vi "Simulation XY update.vi"() -> ()   [LabVIEW 2013]
uses:
  subvi/simulator/Global Variables.vi
panel:
  out "Y Position":dbl
  out "X Position":dbl
  in  "stop":bool
  in  "Update Delay":u32=250
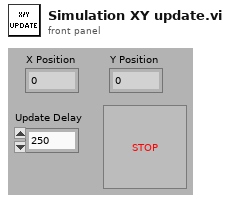
[diagram p1: front panel]
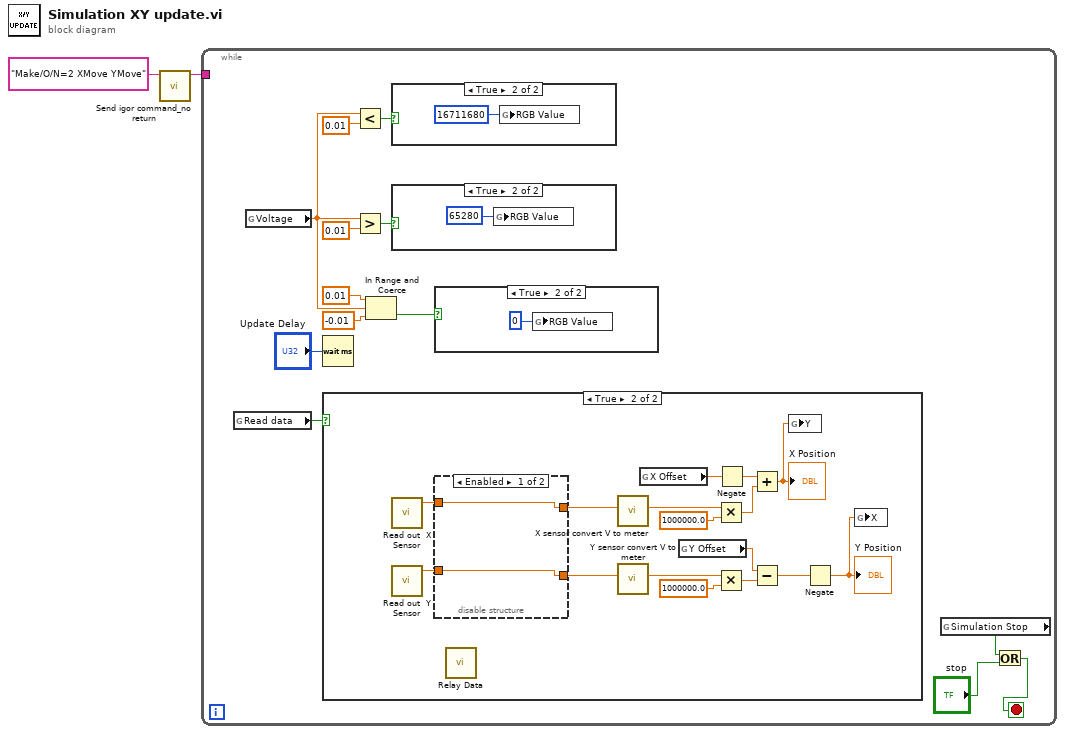
[diagram p0: block diagram]
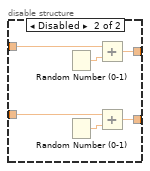
[diagram p6: hidden frame]
diagram:
  n1 = call "Send igor command_no return.vi"("Command"="Make/O/N=2 XMove YMove") -> ("History"=w1:string)  [unwired: 10 out]
  n2 = while {
    tunnel: w1 -> [_]
    stop <- w3 stop-if-true
    n3 = global read "Global Variables.vi" "Read data"() -> (w15:bool)
    n4 = global read "Global Variables.vi" "Voltage"() -> (w6:dbl)
    n5 = Wait (ms)(milliseconds to wait="Update Delay") -> ()  [unwired: 1 out]
    n6 = case shown="True" w15 {
      frame False {
      }
      frame True {
        n7 = call "Read out  X Sensor.vi"() -> ("Result"=w24:dbl)  [unwired: 1 in, 1 out]
        n8 = call "Read out  Y Sensor.vi"() -> ("Result"=w23:dbl)  [unwired: 1 in, 1 out]
        n9 = disable-structure shown="Enabled" {
          disable-tunnel: w23 -> [w35 w42]
          disable-tunnel: w24 -> [w36 w39]
          disable-tunnel: [w36 w38] -> w34
          disable-tunnel: [w35 w37] -> w29
          frame Enabled {
          }
          frame Disabled {
            n10 = Random Number (0-1)() -> (number: 0 to 1=w40:dbl)
            n11 = Random Number (0-1)() -> (number: 0 to 1=w41:dbl)
            n12 = Add(x=w39, y=w40) -> (x+y=w38:dbl)
            n13 = Add(x=w42, y=w41) -> (x+y=w37:dbl)
          }
        }
        n14 = call "Relay Data.vi"() -> ()  [unwired: 12 in]
        n15 = call "X sensor convert V to meter.vi"("Sensor X Voltage"=w34) -> ("X coordinate"=w32:dbl)  [unwired: 10 in]
        n16 = call "Y sensor convert V to meter.vi"("Sensor Y Voltage"=w29) -> ("Y coordinate"=w30:dbl)  [unwired: 10 in]
        n17 = global read "Global Variables.vi" "X Offset"() -> (w22:dbl)
        n18 = global read "Global Variables.vi" "Y Offset"() -> (w21:dbl)
        n19 = Multiply(x=w32, y=1000000.0) -> (x*y=w28:dbl)
        n20 = Multiply(x=w30, y=1000000.0) -> (x*y=w27:dbl)
        n21 = Negate(x=w22) -> (-x=w25:dbl)
        n22 = Add(x=w25, y=w28) -> (x+y=w20:dbl)
        "X Position" <- w20
        n23 = Subtract(x=w21, y=w27) -> (x-y=w26:dbl)
        n24 = global write "Global Variables.vi" "Y"(w20) -> ()
        n25 = Negate(x=w26) -> (-x=w19:dbl)
        "Y Position" <- w19
        n26 = global write "Global Variables.vi" "X"(w19) -> ()
      }
    }
    n27 = Less?(x=w6, y=0.01) -> (x < y?=w10:bool)
    n28 = Greater?(x=w6, y=0.01) -> (0:w12:bool)
    n29 = In Range and Coerce(upper limit=0.01, x=w6, lower limit=-0.01) -> (In Range?=w9:bool)  [unwired: 1 out]
    n30 = case shown="True" w10 {
      frame False {
      }
      frame True {
        n31 = global write "Global Variables.vi" "RGB Value"(16711680) -> ()
      }
    }
    n32 = case shown="True" w12 {
      frame False {
      }
      frame True {
        n33 = global write "Global Variables.vi" "RGB Value"(65280) -> ()
      }
    }
    n34 = case shown="True" w9 {
      frame False {
      }
      frame True {
        n35 = global write "Global Variables.vi" "RGB Value"(0) -> ()
      }
    }
    n36 = global read "Global Variables.vi" "Simulation Stop"() -> (w5:bool)
    n37 = Or(x=w5, y="stop") -> (x .or. y?=w3:bool)
  }
